vi "General Polynomial Fit with SD.vi"(4 "Standard Deviation":dbl[](array[numeric]) format="%.2f", 5 "algorithm":T1(ring), 6 "polynomial order":i32=2, 7 "X Values":dbl[](array[numeric]) format="%.2f", 8 "Y Values":dbl[](array[numeric]) format="%.2f") -> (0 "error":i32, 1 "mse":dbl format="%.2f", 2 "Polynomial Fit Coefficients":dbl[](array[numeric]) format="%.2f", 3 "Best Polynomial Fit":dbl[](array[numeric]) format="%.2f")   [LabVIEW 2011, in "OfflineTracker.lvlib"]
doc: "Finds the polynomial curve values and the set of Polynomial Fit Coefficients, which describe the polynomial curve that best represents the input data set."
uses:
  OfflineTracker.lvlib
  <vilib>/Analysis/NI_AALPro.lvlib
panel:
  # "General Polynomial Fit"
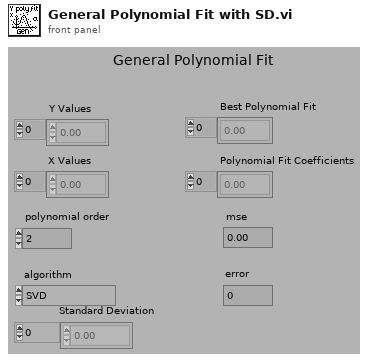
[diagram p1: front panel]
types:
  T1 = enum32{"SVD", "Givens", "Givens2", "Householder", "LU Decomposition", "Cholesky"}
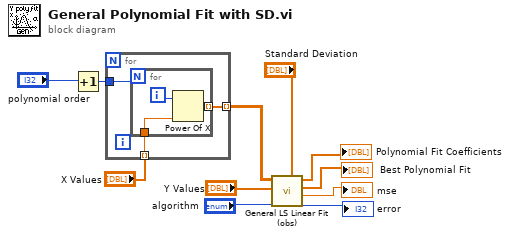
[diagram p0: block diagram]
diagram:
  n1 = Increment(x="polynomial order") -> (x+1=w9:i32)
  n2 = for {
    tunnel: [w14] -> w6 mode=indexing
    tunnel: w9 -> [w13]
    tunnel: "X Values" -> [w12] mode=indexing
    n3 = for {
      N: w13 -> [_]
      tunnel: [w16] -> w14 mode=indexing
      tunnel: w12 -> [w15]
      i -> [w17]
      n4 = Power Of X(1:w15, 2:w17) -> (0:w16:dbl)
    }
  }
  n5 = call <vilib>:"General LS Linear Fit (obs).vi"("H"=w6, "Y"="Y Values", "algorithm"="algorithm", "Standard Deviation"="Standard Deviation") -> ("Coefficients"=→"Polynomial Fit Coefficients":dbl[], "Best Fit"=→"Best Polynomial Fit":dbl[], "mse"=→"mse":dbl, "error"=→"error":i32)  [unwired: 1 in, 1 out]
